vi "array_sort_and_remove_redundancy.vi"(1 "Full Array":u32[](array[numeric])) -> (0 "Non-Redundant Sorted Array":u32[](array[numeric]))   [LabVIEW 2013]
doc: "Takes a 1D array, sorts it, then removes any redundant entries so the output array is always increasing."
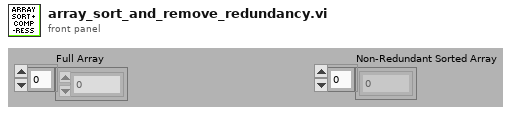
[diagram p1: front panel]
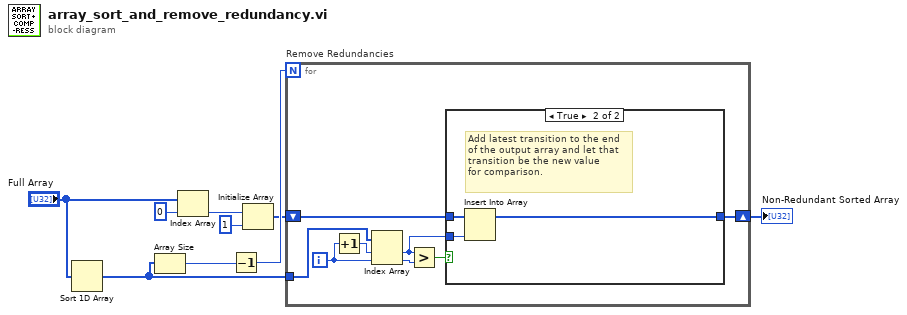
[diagram p0: block diagram]
diagram:
  n1 = Sort 1D Array(array="Full Array") -> (sorted array=w7:u32[])
  n2 = Array Size(array=w7) -> (size(s)=w9:i32)
  n3 = Index Array(array="Full Array", index=0) -> (element=w4:u32)
  n4 = Decrement(x=w9) -> (x-1=w8:i32)
  n5 = Initialize Array(w4, 1 ("dimension size")) -> (w2:u32[])
  n6 = for "Remove Redundancies" {
    N: w8 -> [_]
    shift-right: [w16] -> w1
    shift-left: w2 -> [w17]
    tunnel: w7 -> [w15]
    i -> [w13]
    n7 = Increment(x=w13) -> (x+1=w14:i32)
    n8 = Index Array(array=w15, index #1=w14, index #2=w13) -> (element #1=w10:u32, element #2=w12:u32)
    n9 = Greater?(x=w10, y=w12) -> (0:w11:bool)
    n10 = case shown="True" w11 {
      tunnel: w17 -> [w18 w21]
      tunnel: [w18 w20] -> w16
      tunnel: w10 -> [_ w19]
      frame False {
        # "Add nothing to the output array\nand keep the same value for comparison."
      }
      frame True {
        # "Add latest transition to the end\nof the output array and let that\ntransition be the new value\nfor comparison."
        n11 = Insert Into Array(array=w21, new element=w19) -> (w20:u32[])  [unwired: 1 in]
      }
    }
  }
  "Non-Redundant Sorted Array" <- w1
